vi "BooleanToggle.vi"(9 "InitialState":bool, 11 "Toggle Edge In":bool) -> (1 "Changed":bool, 3 "Output":bool)   [LabVIEW 2023]
uses:
  <vilib>/Rock Robotics/WPI/ThirdParty/JAS_Junk/TrajLib/Trajectory_Library.lvlib
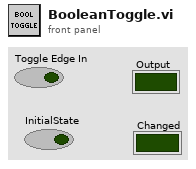
[diagram p1: front panel]
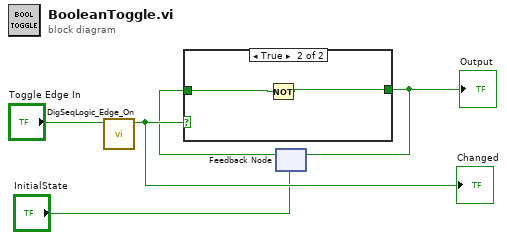
[diagram p0: block diagram]
diagram:
  n1 = call <vilib>:"DigSeqLogic_Edge_On.vi"("Input"="Toggle Edge In") -> ("On Edge"=w3:bool)  [unwired: 10 in]
  "Changed" <- w3
  n2 = feedback #1("InitialState") -> (w1:bool)
  n3 = case shown="True" w3 {
    tunnel: w1 -> [w6 w8]
    tunnel: [w6 w7] -> w5
    frame False {
    }
    frame True {
      n4 = Not(x=w8) -> (.not. x?=w7:bool)
    }
  }
  "Output" <- w5
  n5 = feedback-in #1(w5) -> ()
